vi "Insert Reserved Error.vi"(3 "Insert as Warning? (False: Insert as Error)":bool, 4 "error in (no error)":errorcluster, 5 "error description":string, 6 "Reserved Error Code (Generic error)":u16(ring)=42 items=["No error", "Argument error", "Memory is full", "Out of zone", "End of file", "File already open", "Generic file I/O error", "File not found", "File permission error", "Disk is full", "Duplicate path", "Too many files open", "System feature not enabled", "Resource file not found", "Cannot add resource", "Resource not found", "Image not found", "Image memory error", "Pen does not exist", "Config type invalid", "Config token not found", "Config parse error", "Config memory error", "Bad external code format", "Bad external code offset", "External code not present", "Null window", "Destroy window error", "Null menu", "Print aborted", "Bad print record", "Print driver error", "Windows error during printing", "Memory error during printing", "Print dialog error", "Generic print error", "Invalid device refnum", "Device not found", "Device parameter error", "Device unit error", "Cannot open device", "Device call aborted", "Generic error", "Cancelled by user", "Object ID too low", "Object ID too high", "Object not in heap", "Unknown heap", "Unknown object (invalid DefProc)", "Unknown object (DefProc not in table)", "Message out of range", "Invalid (null) method", "Unknown message", "Manager call not supported", "Bad address", "Network operation in progress", "Network operation timed out", "Connection is busy", "Network attribute not supported", "Network error", "Address in use", "System out of memory", "Connection aborted", "Connection refused", "Not connected", "Already connected", "Connection closed", "Initialization error (interapplication manager)", "Bad occurrence", "Wait on unbound occurrence handler", "Occurrence queue overflow", "Datalog type conflict", "Unused", "Unrecognized type (interapplication manager)", "Memory corrupt", "Failed to make temporary DLL", "Old CIN version", "Drag socket not found", "Failed to load drop-object", "Failed to register OLE object", "Failed to release OLE object", "Format specifier type mismatch", "Unknown format specifier", "Too few format specifiers", "Too many format specifiers", "Scan failed", "Newer CIN version", "OLE Convert", "Runtime menu error", "Password tampered", "Unknown error code"], 7 "error? (True)":bool=TRUE) -> (0 "error out":errorcluster)   [LabVIEW 2013]
doc: "Wire \"Reserved error code\" with an error ring constant to be inserted unless there's an upstream error or \"error?\" is false. Source string is built from the calling chain, starting with this vi's caller, and prepended with \"error description\" input.\n\nFreeware from Moore Good Ideas, www.mooregoodideas.com. Do not remove this line."
panel:
  in  "call chain header":string="\n<b>Complete call chain:</b>"
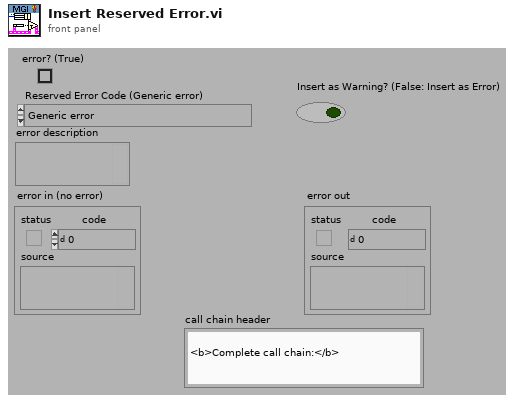
[diagram p1: front panel]
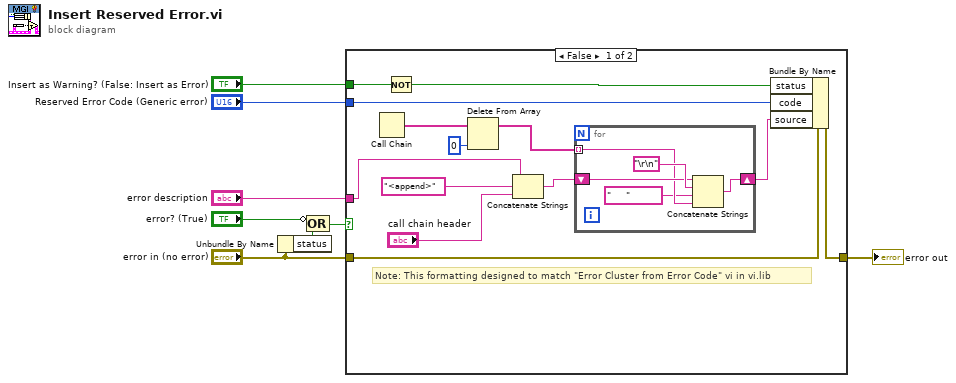
[diagram p0: block diagram]
diagram:
  n1 = Unbundle By Name("error in (no error)") -> ("status"=w3:bool)
  n2 = Compound Arithmetic op=OR(invert "error? (True)", w3) -> (w2:bool)
  n3 = case shown="False" w2 {
    tunnel: "error in (no error)" -> [w21 w27]
    tunnel: [w20 w27] -> w6
    tunnel: "error description" -> [w11 _]
    tunnel: "Reserved Error Code (Generic error)" -> [w19 _]
    tunnel: "Insert as Warning? (False: Insert as Error)" -> [w10 _]
    frame False {
      # "Note: This formatting designed to match \"Error Cluster from Error Code\" vi in vi.lib"
      n4 = Call Chain() -> (call chain=w13:string[])
      n5 = Not(x=w10) -> (.not. x?=w9:bool)
      n6 = Delete From Array(array=w13, index=0) -> (array with subset deleted=w14:string[])  [unwired: 1 in, 1 out]
      n7 = Concatenate Strings(w11, "<append>", "call chain header") -> (w17:string)
      n8 = for {
        tunnel: w14 -> [w23] mode=indexing
        shift-right: [w26] -> w12
        shift-left: w17 -> [w24]
        n9 = Concatenate Strings(w24, "\r\n", "     ", w23) -> (w26:string)
      }
      n10 = Bundle By Name(cluster=w21, "status"=w9, "code"=w19, "source"=w12) -> (w20:errorcluster)
    }
    frame True {
    }
  }
  "error out" <- w6
